vi "dynamatic.vi"(8 "error in (no error)":errorcluster, 11 "IChildFoo in":refnum<class "IChildFoo.lvclass">) -> (0 "error out":errorcluster, 3 "IChildFoo out":refnum<class "IChildFoo.lvclass">)   [LabVIEW 2021, in "IChildFoo.lvclass"]
uses:
  IChildFoo.lvclass
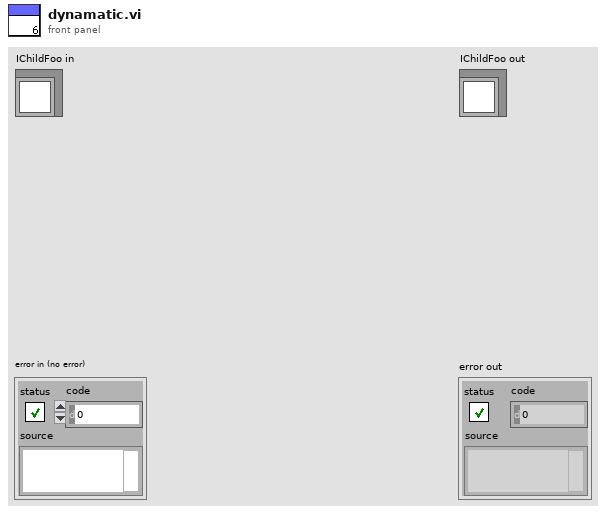
[diagram p1: front panel]
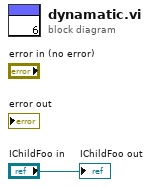
[diagram p0: block diagram]
diagram:
  "IChildFoo out" <- "IChildFoo in"
